vi "Setup TS.vi"(8 "error in":errorcluster, 11 "LNG Boiling Test Stand in":refnum<class "LNG Boiling Test Stand.lvclass">) -> (0 "error out":errorcluster, 3 "LNG Boiling Test Stand out":refnum<class "LNG Boiling Test Stand.lvclass">)   [LabVIEW 2019, in "Test Stands.lvlib" / "LNG Boiling Test Stand.lvclass"]
uses:
  LNG Boiling Test Stand.lvclass
  C:/Users/krio/Documents/LV_Projects/test-stand/App/Generic Test Stand/Generic Test Stand.lvclass
  DAC/LNG Boiling/Heater Box Temperatures/DAC Heater Box Temperatures.lvclass
  C:/Users/krio/Documents/LV_Projects/test-stand/App/DAC/DAC.lvclass
  DAC/DAC.lvclass
  DAC/LNG Boiling/Shunt dU/DAC Shunt dU.lvclass
  DAC/LNG Boiling/Heater dU/DAC Heater dU.lvclass
  DAC/LNG Boiling/Heater Ctrl/DAC Heater Ctrl.lvclass
  DAC/DAC.lvclass/DAC.ctl
  Generic Test Stand/Generic Test Stand.lvclass/Generic Test Stand.ctl
  Generic Test Stand/Generic Test Stand.lvclass
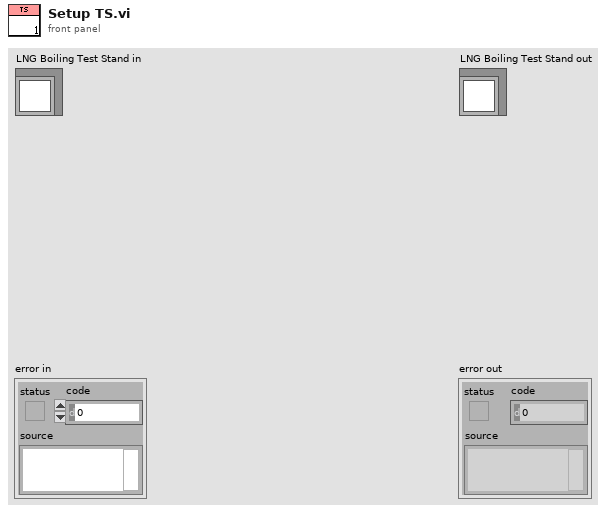
[diagram p1: front panel]
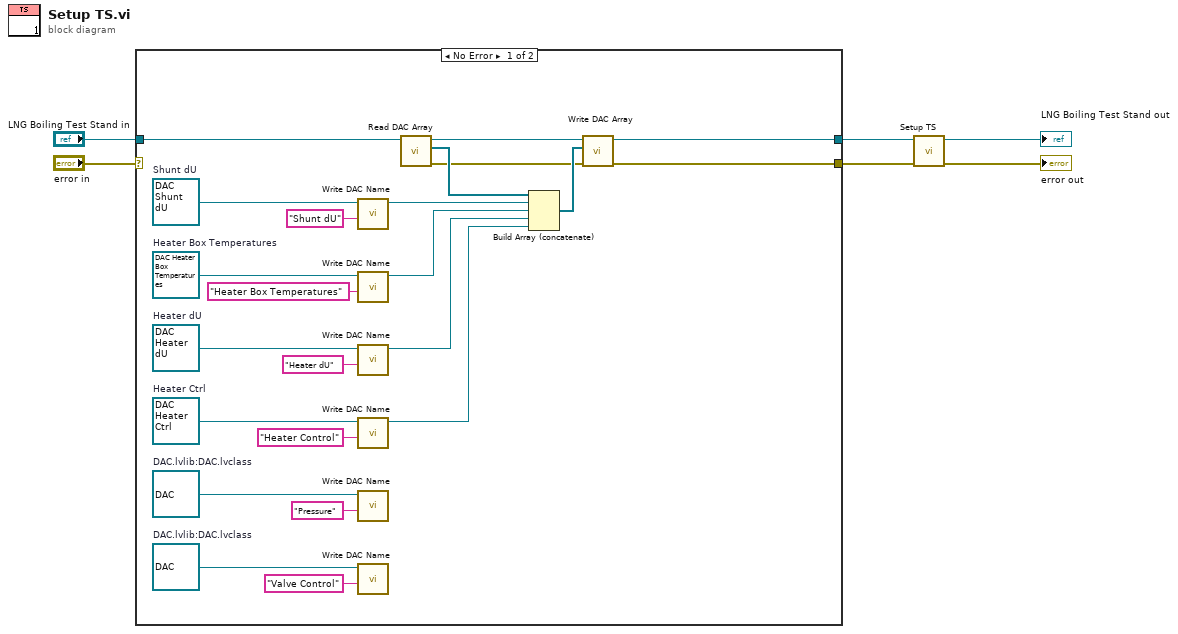
[diagram p0: block diagram]
diagram:
  n1 = case shown="No Error" "error in" {
    selector: "error in" -> [_ w30]
    tunnel: "LNG Boiling Test Stand in" -> [w28 w31]
    tunnel: [w8 w31] -> w2
    tunnel: [w7 w30] -> w1
    frame No Error {
      w15 = refnum<class "DAC Heater Ctrl.lvclass"> refnum  # Heater Ctrl
      w17 = refnum<class "DAC Heater dU.lvclass"> refnum  # Heater dU
      w19 = refnum<class "DAC Shunt dU.lvclass"> refnum  # Shunt dU
      w20 = refnum<class "DAC.lvclass"> refnum  # DAC.lvlib:DAC.lvclass
      w21 = refnum<class "DAC.lvclass"> refnum  # DAC.lvlib:DAC.lvclass
      w29 = refnum<class "DAC Heater Box Temperatures.lvclass"> refnum  # Heater Box Temperatures
      n2 = call "Write DAC Name.vi"("DAC Name"="Shunt dU", "DAC in"=w19) -> ("DAC out"=w23:refnum<class "DAC Shunt dU.lvclass">)  [unwired: 8 in, 1 out]
      n3 = call "Write DAC Name.vi"("DAC Name"="Heater Box Temperatures", "DAC in"=w29) -> ("DAC out"=w22:refnum<class "DAC Heater Box Temperatures.lvclass">)  [unwired: 8 in, 1 out]
      n4 = call "Write DAC Name.vi"("DAC Name"="Heater dU", "DAC in"=w17) -> ("DAC out"=w18:refnum<class "DAC Heater dU.lvclass">)  [unwired: 8 in, 1 out]
      n5 = call "Write DAC Name.vi"("DAC Name"="Heater Control", "DAC in"=w15) -> ("DAC out"=w16:refnum<class "DAC Heater Ctrl.lvclass">)  [unwired: 8 in, 1 out]
      n6 = call "Write DAC Name.vi"("DAC Name"="Pressure", "DAC in"=w21) -> ()  [unwired: 8 in, 2 out]
      n7 = call "Write DAC Name.vi"("DAC Name"="Valve Control", "DAC in"=w20) -> ()  [unwired: 8 in, 2 out]
      n8 = call "Read DAC Array.vi"("Generic Test Stand in"=w28) -> ("error out"=w24:errorcluster, "DAC Array"=w27:refnum<class "DAC.lvclass">[], "Generic Test Stand out"=w26:refnum<class "LNG Boiling Test Stand.lvclass">)  [unwired: 8 in]
      n9 = Build Array (concatenate)(w27, w23, w22, w18, w16) -> (w25:refnum<class "DAC.lvclass">[])
      n10 = call "Write DAC Array.vi"("error in (no error)"=w24, "DAC Array"=w25, "Generic Test Stand in"=w26) -> ("error out"=w7:errorcluster, "Generic Test Stand out"=w8:refnum<class "LNG Boiling Test Stand.lvclass">)  [unwired: 7 in]
    }
    frame Error {
    }
  }
  n11 = call-parent "Setup TS.vi"("error in (no error)"=w1, "Generic Test Stand in"=w2) -> ("error out"=→"error out":errorcluster, "Generic Test Stand out"=→"LNG Boiling Test Stand out":refnum<class "LNG Boiling Test Stand.lvclass">)  [unwired: 8 in]
